vi "Generate Callchain.vi"() -> (3 "Callchain":string)   [LabVIEW 2016, in "hse-logger.lvlib" / "LogRecord.lvclass"]
doc: "Generates a easy to read callchain. Entries from the hse-logger.lvlib are ignored."
uses:
  LogRecord.lvclass
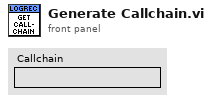
[diagram p1: front panel]
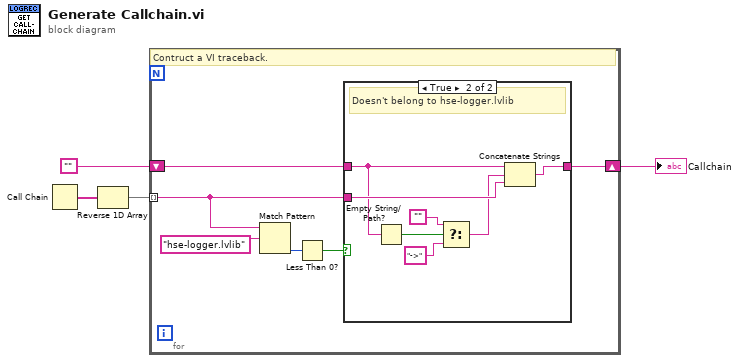
[diagram p0: block diagram]
diagram:
  n1 = Call Chain() -> (call chain=w2:string[])
  n2 = Reverse 1D Array(array=w2) -> (reversed array=w1:string[])
  n3 = for {
    tunnel: w1 -> [w5] mode=indexing
    shift-right: [w9] -> w4
    shift-left: "" -> [w10]
    # "Contruct a VI traceback."
    n4 = Match Pattern(string=w5, regular expression="hse-logger.lvlib") -> (offset past match=w7:i32)  [unwired: 1 in, 3 out]
    n5 = Less Than 0?(x=w7) -> (x < 0?=w6:bool)
    n6 = case shown="True" w6 {
      tunnel: w10 -> [w11 w16]
      tunnel: [w11 w18] -> w9
      tunnel: w5 -> [_ w17]
      frame False {
        # "hse-logger.lvlib entry, don't add\nit to the callchain."
      }
      frame True {
        # "Doesn't belong to hse-logger.lvlib"
        n7 = Empty String/Path?(string/path=w16) -> (empty?=w15:bool)
        n8 = Select(t="", s=w15, f="->") -> (s? t:f=w14:string)
        n9 = Concatenate Strings(w16, w14, w17) -> (w18:string)
      }
    }
  }
  "Callchain" <- w4
